vi "set_position.vi"(8 "error in (no error)":errorcluster, 10 "new position":dbl, 11 "ESP301_via_TCPIP in":refnum<class "ESP301_via_TCPIP.lvclass">) -> (0 "error out":errorcluster, 3 "ESP301_via_TCPIP out":refnum<class "ESP301_via_TCPIP.lvclass">)   [LabVIEW 2018, in "ESP301_via_TCPIP.lvclass"]
uses:
  ESP301_via_TCPIP.lvclass
  _delayStageBase/_delayStageBase.lvclass
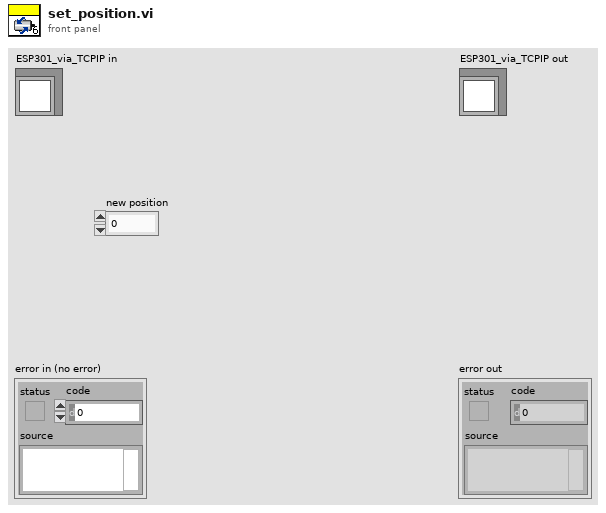
[diagram p1: front panel]
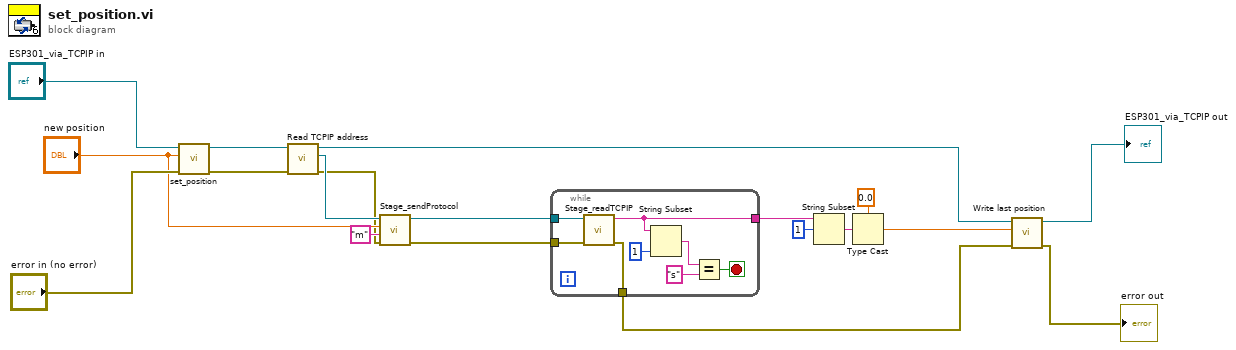
[diagram p0: block diagram]
diagram:
  n1 = call-parent "set_position.vi"("error in (no error)"="error in (no error)", "last position"="new position", "_delayStageBase in"="ESP301_via_TCPIP in") -> ("error out"=w15:errorcluster, "_delayStageBase out"=w14:refnum<class "ESP301_via_TCPIP.lvclass">)  [unwired: 7 in]
  n2 = call-dynamic "Read TCPIP address.vi"("error in (no error)"=w15, "ESP301_via_TCPIP in"=w14) -> ("error out"=w12:errorcluster, "TCPIP address"=w13:refnum<k5>, "ESP301_via_TCPIP out"=w5:refnum<class "ESP301_via_TCPIP.lvclass">)  [unwired: 7 in]
  n3 = call "Stage_sendProtocol.vi"("error in (no error)"=w12, "command"="m", "GoTo position"="new position", "TCP Network Connection in"=w13) -> ("error out"=w2:errorcluster, "TCP Network Connection out"=w11:refnum<k5>)  [unwired: 6 in]
  n4 = while {
    tunnel: w11 -> [w27]
    tunnel: [w24] -> w10
    tunnel: w2 -> [w21]
    tunnel: [w20] -> w1
    stop <- w25 stop-if-true
    n5 = call "Stage_readTCPIP.vi"("error in (no error)"=w21, "TCP Network Connection in"=w27) -> ("error out"=w20:errorcluster, "data out"=w24:string)  [unwired: 8 in]
    n6 = String Subset(string=w24, length (rest)=1 ("offset (0)")) -> (substring=w22:string)  [unwired: 1 in]
    n7 = Equal?(x=w22, y="s") -> (x = y?=w25:bool)
  }
  n8 = String Subset(string=w10, offset (0)=1) -> (substring=w8:string)  [unwired: 1 in]
  n9 = Type Cast(type=0.0, x=w8) -> (*(type *) &x=w6:dbl)
  n10 = call-dynamic "Write last position.vi"("error in (no error)"=w1, "last position"=w6, "_delayStageBase in"=w5) -> ("error out"=→"error out":errorcluster, "_delayStageBase out"=→"ESP301_via_TCPIP out":refnum<class "ESP301_via_TCPIP.lvclass">)  [unwired: 7 in]
